vi "Check for Timeout.vi"(7 "Timeout(S)":dbl=1.5, 8 "error in (no error)":errorcluster, 11 "Start Time":timestamp) -> (0 "error out":errorcluster)   [LabVIEW 2019, in "Network Messenger.lvlib" / "ReadStrategy.lvclass"]
uses:
  <vilib>/gpm_packages/@cs/Network-interface/Source/Network Messenger/ReadStrategy/ReadStrategy.lvclass
  <vilib>/Utility/error.llb/Error Cluster From Error Code.vi
  <vilib>/ErrorRing/Error Ring.xnode
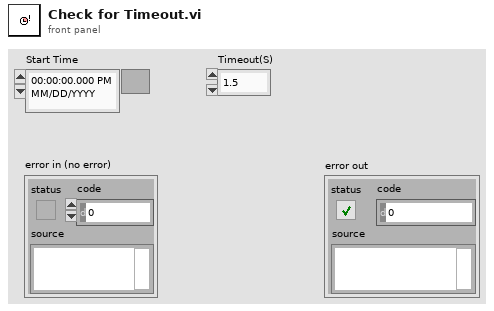
[diagram p1: front panel]
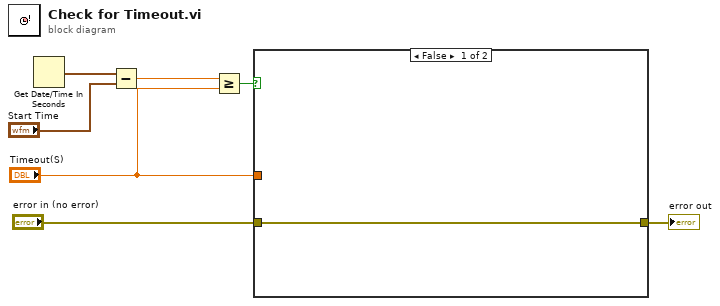
[diagram p0: block diagram]
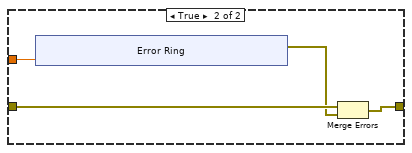
[diagram p2: hidden frame]
diagram:
  n1 = Get Date/Time In Seconds() -> (seconds since 1Jan1904=w7:timestamp)
  n2 = Subtract(x=w7, y="Start Time") -> (x-y=w5:dbl)
  n3 = Greater Or Equal?(x=w5, y="Timeout(S)") -> (x >= y?=w4:bool)
  n4 = case shown="False" w4 {
    tunnel: "error in (no error)" -> [w8 w12]
    tunnel: "Timeout(S)" -> [_ w11]
    tunnel: [w8 w10] -> w1
    frame False {
    }
    frame True {
      n5 = xnode "Error Ring"("parameter 0"=w11) -> ("error out"=w9:errorcluster)
      n6 = Merge Errors(w12, w9) -> (w10:errorcluster)
    }
  }
  "error out" <- w1
